vi "USRP TX.vi"() -> ()   [LabVIEW 2022 SP3]
uses:
  <instrlib>/niUSRP/niUSRP Write Tx Data (CDB).vi
panel:
  in  "end of data?":bool
  out "coerced gain":dbl format="%#_6f"
  out "coerced carrier frequency":dbl=100000.0 format="%#_6p"
  out "coerced IQ rate":dbl=100000.0 format="%#_6p"
  in  "active antenna":string
  in  "gain":dbl format="%#_6f"
  in  "carrier frequency":dbl=100000.0 format="%#_6p"
  in  "IQ rate":dbl=100000.0 format="%#_6p"
  out "error out":errorcluster
  in  "device names":refnum<k15>
  in  "waveform size":i32
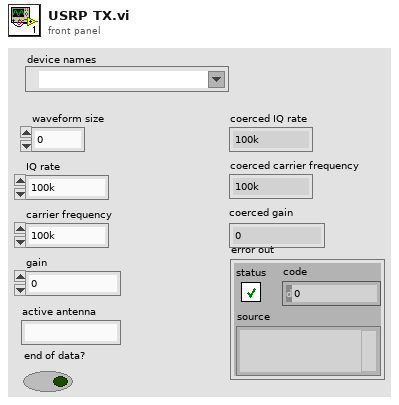
[diagram p1: front panel]
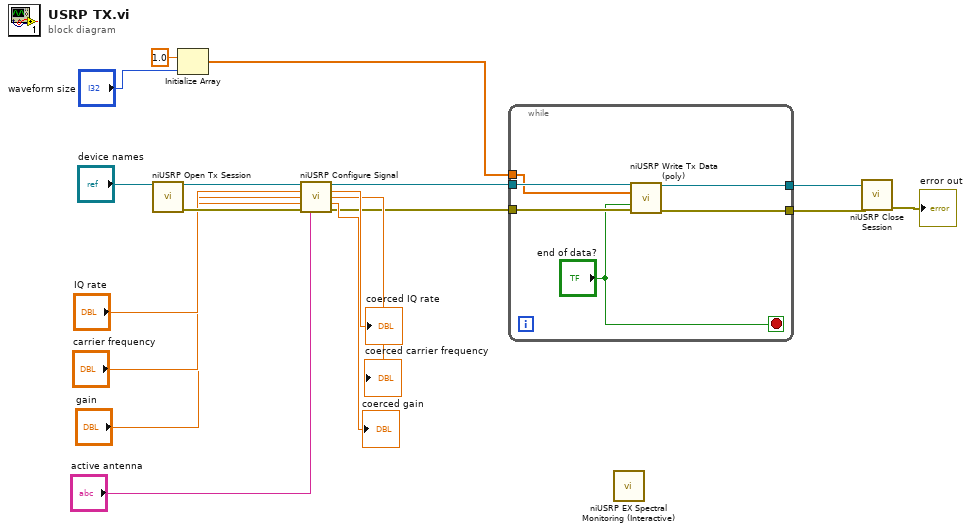
[diagram p0: block diagram]
diagram:
  n1 = call <instrlib>:"niUSRP Open Tx Session.vi"("device names"="device names") -> ("session handle out"=w17:refnum<k15>, "error out"=w16:errorcluster)  [unwired: 13 in]
  n2 = Initialize Array(1.0 ("element"), "waveform size") -> (w5:dbl[])
  n3 = call <instrlib>:"niUSRP Configure Signal.vi"("session handle"=w17, "IQ rate"="IQ rate", "carrier frequency"="carrier frequency", "gain"="gain", "error in (no error)"=w16, "active antenna"="active antenna") -> ("session handle out"=w4:refnum<k15>, "coerced IQ rate"=→"coerced IQ rate":dbl, "coerced carrier frequency"=→"coerced carrier frequency":dbl, "coerced gain"=→"coerced gain":dbl, "error out"=w2:errorcluster)  [unwired: 5 in]
  n4 = while {
    tunnel: w5 -> [w23]
    tunnel: w4 -> [w24]
    tunnel: [w22] -> w3
    tunnel: w2 -> [w21]
    tunnel: [w20] -> w1
    stop <- "end of data?" stop-if-true
    n5 = call-poly <instrlib>:"niUSRP Write Tx Data (poly).vi"("session handle"=w24, "data"=w23, "end of data?"="end of data?", "error in (no error)"=w21) -> ("session handle out"=w22:refnum<k15>, "error out"=w20:errorcluster)  [unwired: 10 in]
  }
  n6 = call "niUSRP EX Spectral Monitoring (Interactive).vi"() -> ()  [unwired: 1 in]
  n7 = call <instrlib>:"niUSRP Close Session.vi"("session handle"=w3, "error in (no error)"=w1) -> ("error out"=→"error out":errorcluster)  [unwired: 13 in]
